vi "calc_move.vi"(2 "z":dbl format="%#_13g", 3 "y":dbl format="%#_13g", 4 "Numeric":i32, 5 "x":dbl format="%#_13g") -> (0 "x-y":dbl)   [LabVIEW 2017]
uses:
  <vilib>/Analysis/Matrix/Datatypes/RealMatrix.ctl
  Downloads/LinRS_ZIEMIECKI/PRZEDOSTATECZNA_WERSJA/LinRS_connect/Pozycja_dol.ctl
  Downloads/LinRS_ZIEMIECKI/PRZEDOSTATECZNA_WERSJA/LinRS_connect/Pozycja_gora.ctl
  <vilib>/Analysis/Matrix/Numeric/Conversions/Array To Matrix - RA.vi
  <vilib>/Analysis/Matrix/Numeric/Conversions/Array To Matrix - RA2.vi
  <vilib>/Analysis/Matrix/Numeric/Add/Add - RM,RM.vi
  <vilib>/Analysis/Matrix/Numeric/Multiply/Multiply - RM,RM.vi
  <vilib>/Analysis/Matrix/Numeric/Conversions/Matrix To Array - RM.vi
  <vilib>/Analysis/Matrix/NI_Matrix.lvlib
panel:
  out "A + B 2":T1
  out "A + B":T1
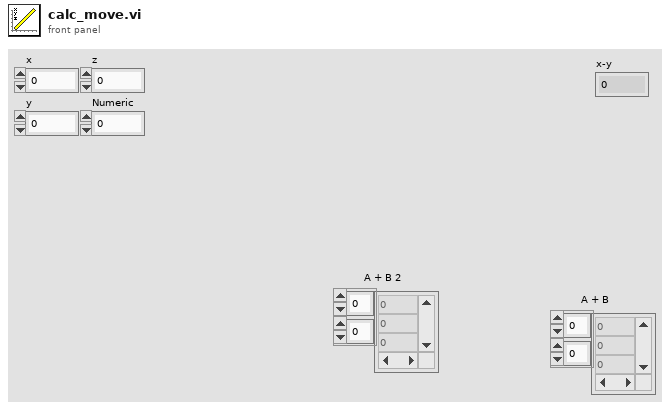
[diagram p1: front panel]
types:
  T1 = typedef "NI_Matrix.lvlib/RealMatrix.ctl" = dbl[][]
  T2 = typedef "Pozycja_zero.ctl" = sgl[][]
  T3 = typedef "Pozycja_gora.ctl" = sgl[][]
  T4 = typedef "Pozycja_dol.ctl" = sgl[][]
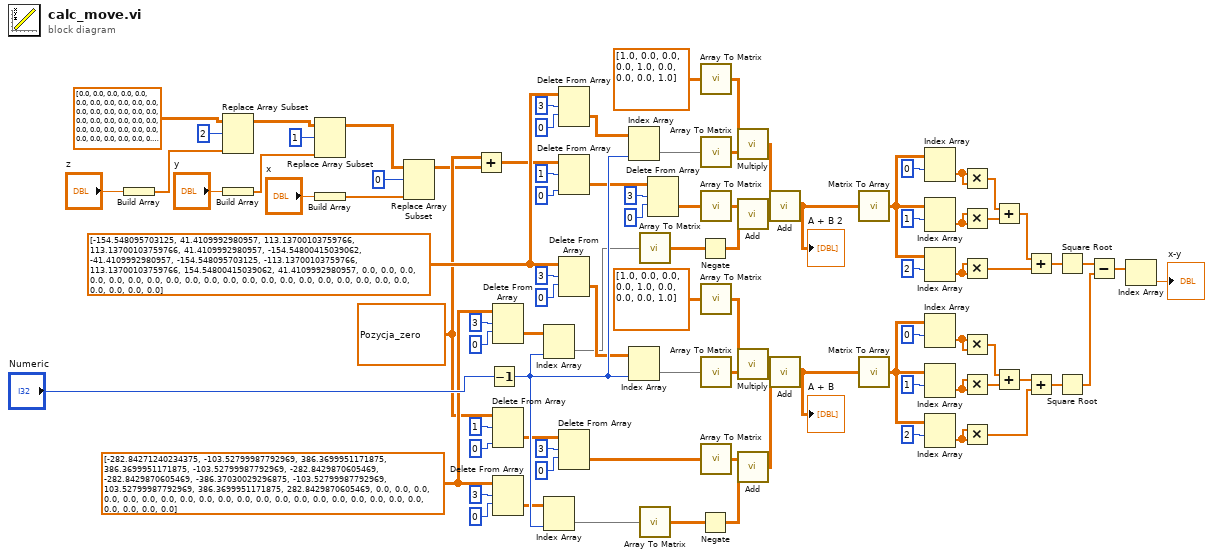
[diagram p0: block diagram]
diagram:
  w22 = T2 [[0.0, 0.0, 0.0, 0.0, 0.0, 0.0], [0.0, 0.0, 0.0, 0.0, 0.0, 0.0], [644.23, 0.0, 0.0, 0.0, 0.0, 0.0], [0.0, 0.0, 0.0, 0.0, 0.0, 0.0], [0.0, 0.0, 0.0, 0.0, 0.0, 0.0], [0.0, 0.0, 0.0, 0.0, 0.0, 0.0]]
  w24 = T3 [[-154.5481, 41.411, 113.137, 113.137, 41.411, -154.548], [-41.411, -154.5481, -113.137, 113.137, 154.548, 41.411], [0.0, 0.0, 0.0, 0.0, 0.0, 0.0], [0.0, 0.0, 0.0, 0.0, 0.0, 0.0], [0.0, 0.0, 0.0, 0.0, 0.0, 0.0], [0.0, 0.0, 0.0, 0.0, 0.0, 0.0]]
  w23 = T4 [[-282.8427, -103.528, 386.37, 386.37, -103.528, -282.843], [-282.843, -386.3703, -103.528, 103.528, 386.37, 282.843], [0.0, 0.0, 0.0, 0.0, 0.0, 0.0], [0.0, 0.0, 0.0, 0.0, 0.0, 0.0], [0.0, 0.0, 0.0, 0.0, 0.0, 0.0], [0.0, 0.0, 0.0, 0.0, 0.0, 0.0]]
  n1 = Build Array("z") -> (w15:dbl[])
  n2 = Replace Array Subset(array=sgl[][] [[0.0, 0.0, 0.0, 0.0, 0.0, 0.0], [0.0, 0.0, 0.0, 0.0, 0.0, 0.0], [0.0, 0.0, 0.0, 0.0, 0.0, 0.0], [0.0, 0.0, 0.0, 0.0, 0.0, 0.0], [0.0, 0.0, 0.0, 0.0, 0.0, 0.0], [0.0, 0.0, 0.0, 0.0, 0.0, 0.0]], new element=w15, index (row)=2) -> (w17:sgl[][])  [unwired: 1 in]
  n3 = Build Array("y") -> (w16:dbl[])
  n4 = Replace Array Subset(array=w17, new element=w16, index (row)=1) -> (w18:sgl[][])  [unwired: 1 in]
  n5 = Build Array("x") -> (w19:dbl[])
  n6 = Replace Array Subset(array=w18, new element=w19, index (row)=0) -> (w20:sgl[][])  [unwired: 1 in]
  n7 = Add(x=w22, y=w20) -> (x+y=w21:T2)
  n8 = Decrement(x="Numeric") -> (x-1=w92:i32)
  n9 = Delete From Array(array=w23, length=3, index (row)=0) -> (deleted portion=w25:T4)  [unwired: 1 in, 1 out]
  n10 = Delete From Array(array=w22, length=1, index (col)=0 ("disabled index (col)")) -> (deleted portion=w85:T2)  [unwired: 1 in, 1 out]
  n11 = Delete From Array(array=w23, length=3, index (row)=0) -> (deleted portion=w82:T4)  [unwired: 1 in, 1 out]
  n12 = Index Array(array=w25, index (col)=w92) -> (element=w39:sgl[])  [unwired: 1 in]
  n13 = Index Array(array=w82, index (col)=w92) -> (element=w77:sgl[])  [unwired: 1 in]
  n14 = Delete From Array(array=w24, length=3, index (row)=0) -> (deleted portion=w35:T3)  [unwired: 1 in, 1 out]
  n15 = Delete From Array(array=w21, length=1, index (col)=0 ("disabled index (col)")) -> (deleted portion=w32:T2)  [unwired: 1 in, 1 out]
  n16 = Delete From Array(array=w24, length=3, index (row)=0) -> (deleted portion=w81:T3)  [unwired: 1 in, 1 out]
  n17 = Delete From Array(array=w85, length=3, index (row)=0 ("disabled index (col)")) -> (deleted portion=w78:T2)  [unwired: 1 in, 1 out]
  n18 = Index Array(array=w35, index (col)=w92) -> (element=w37:sgl[])  [unwired: 1 in]
  n19 = Index Array(array=w81, index (col)=w92) -> (element=w79:sgl[])  [unwired: 1 in]
  n20 = call-poly <vilib>:"Array To Matrix.vi"("Real 1D Array"=w39) -> ("Real Matrix (Column Vector)"=w40:T1)
  n21 = call-poly <vilib>:"Array To Matrix.vi"("Real 1D Array"=w77) -> ("Real Matrix (Column Vector)"=w76:T1)
  n22 = Delete From Array(array=w32, length=3, index (row)=0 ("disabled index (col)")) -> (deleted portion=w38:T2)  [unwired: 1 in, 1 out]
  n23 = Negate(x=w40) -> (-x=w41:T1)
  n24 = Negate(x=w76) -> (-x=w75:T1)
  n25 = call-poly <vilib>:"Array To Matrix.vi"("Real 2D Array"=sgl[][] [[1.0, 0.0, 0.0], [0.0, 1.0, 0.0], [0.0, 0.0, 1.0]] ("Numeric")) -> ("Real Matrix"=w44:T1)
  n26 = call-poly <vilib>:"Array To Matrix.vi"("Real 1D Array"=w37) -> ("Real Matrix (Column Vector)"=w45:T1)
  n27 = call-poly <vilib>:"Array To Matrix.vi"("Real 2D Array"=w38) -> ("Real Matrix"=w42:T1)
  n28 = call-poly <vilib>:"Array To Matrix.vi"("Real 2D Array"=sgl[][] [[1.0, 0.0, 0.0], [0.0, 1.0, 0.0], [0.0, 0.0, 1.0]] ("Numeric")) -> ("Real Matrix"=w72:T1)
  n29 = call-poly <vilib>:"Array To Matrix.vi"("Real 1D Array"=w79) -> ("Real Matrix (Column Vector)"=w71:T1)
  n30 = call-poly <vilib>:"Array To Matrix.vi"("Real 2D Array"=w78) -> ("Real Matrix"=w74:T1)
  n31 = call-poly <vilib>:"Multiply.vi"("Real Matrix B"=w45, "Real Matrix A"=w44) -> ("A * B"=w46:T1)
  n32 = call-poly <vilib>:"Add.vi"("Real Matrix B"=w41, "Real Matrix A"=w42) -> ("A + B"=w43:T1)
  n33 = call-poly <vilib>:"Multiply.vi"("Real Matrix B"=w71, "Real Matrix A"=w72) -> ("A * B"=w70:T1)
  n34 = call-poly <vilib>:"Add.vi"("Real Matrix B"=w75, "Real Matrix A"=w74) -> ("A + B"=w73:T1)
  n35 = call-poly <vilib>:"Add.vi"("Real Matrix B"=w43, "Real Matrix A"=w46) -> ("A + B"=w2:T1)
  "A + B 2" <- w2
  n36 = call-poly <vilib>:"Add.vi"("Real Matrix B"=w73, "Real Matrix A"=w70) -> ("A + B"=w4:T1)
  "A + B" <- w4
  n37 = call-poly <vilib>:"Matrix To Array.vi"("Real Matrix"=w2) -> ("Real 2D Array"=w47:dbl[][])
  n38 = call-poly <vilib>:"Matrix To Array.vi"("Real Matrix"=w4) -> ("Real 2D Array"=w5:dbl[][])
  n39 = Index Array(array=w47, index (row)=0 ("length")) -> (element=w51:dbl[])  [unwired: 1 in]
  n40 = Index Array(array=w47, index (row)=1 ("length")) -> (element=w52:dbl[])  [unwired: 1 in]
  n41 = Index Array(array=w47, index (row)=2 ("length")) -> (element=w53:dbl[])  [unwired: 1 in]
  n42 = Index Array(array=w5, index (row)=0 ("length")) -> (element=w66:dbl[])  [unwired: 1 in]
  n43 = Index Array(array=w5, index (row)=1 ("length")) -> (element=w65:dbl[])  [unwired: 1 in]
  n44 = Index Array(array=w5, index (row)=2 ("length")) -> (element=w64:dbl[])  [unwired: 1 in]
  n45 = Multiply(x=w51, y=w51) -> (x*y=w54:dbl[])
  n46 = Multiply(x=w52, y=w52) -> (x*y=w55:dbl[])
  n47 = Multiply(x=w53, y=w53) -> (x*y=w57:dbl[])
  n48 = Multiply(x=w66, y=w66) -> (x*y=w63:dbl[])
  n49 = Multiply(x=w65, y=w65) -> (x*y=w62:dbl[])
  n50 = Multiply(x=w64, y=w64) -> (x*y=w60:dbl[])
  n51 = Add(x=w54, y=w55) -> (x+y=w56:dbl[])
  n52 = Add(x=w63, y=w62) -> (x+y=w61:dbl[])
  n53 = Add(x=w56, y=w57) -> (x+y=w58:dbl[])
  n54 = Add(x=w61, y=w60) -> (x+y=w59:dbl[])
  n55 = Square Root(x=w58) -> (sqrt(x)=w1:dbl[])
  n56 = Square Root(x=w59) -> (sqrt(x)=w3:dbl[])
  n57 = Subtract(x=w1, y=w3) -> (x-y=w7:dbl[])
  n58 = Index Array(array=w7) -> (element=→"x-y":dbl)  [unwired: 1 in]
